vi "Select Active Channels.vi"(8 "error in (no error)":errorcluster, 10 "Active Channel(s)":T1[](array[typedef]), 11 "DPO4104 in":refnum<class "DPO4104.lvclass">) -> (0 "error out":errorcluster, 3 "DPO4104 out":refnum<class "DPO4104.lvclass">)   [LabVIEW 2018, in "DPO4104.lvlib" / "DPO4104.lvclass"]
doc: "This Override method is used to set active channels for the Oscope. Use the 'Active Channel(s)' control to select channel(s)."
uses:
  DPO4104.lvclass
  PPLs/Oscilloscope/Parent/Oscilloscope.lvlibp/Custom Controls/Analog Channels.ctl
  PPLs/Oscilloscope/Parent/Oscilloscope.lvlibp/Oscilloscope.lvclass
  C:/Projects/LabVIEW/PPLs/Oscilloscope/Parent/Oscilloscope.lvlibp/Oscilloscope.lvclass
  PPLs/Oscilloscope/Parent/Oscilloscope.lvlibp
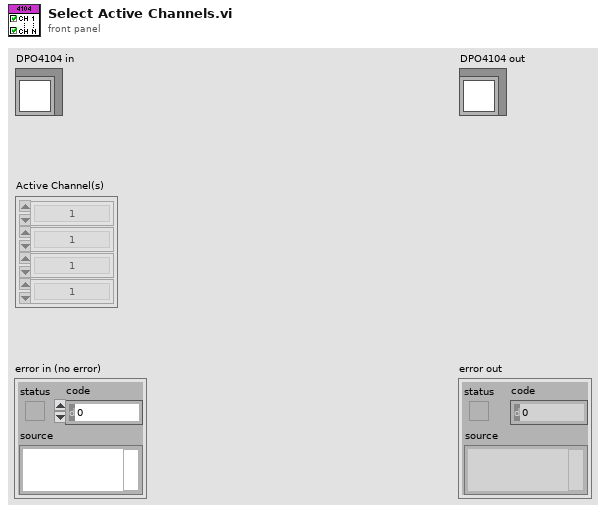
[diagram p1: front panel]
types:
  T1 = typedef "Oscilloscope.lvlibp/Analog Channels.ctl" = enum16{"1", "2", "3", "4", "5", "6", "7", "8", "9", "10", "11", "12", "13", "14", "15", "16"}
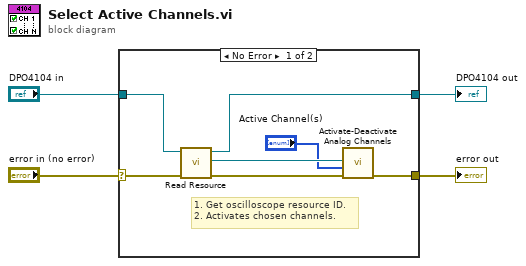
[diagram p0: block diagram]
diagram:
  n1 = case shown="No Error" "error in (no error)" {
    selector: "error in (no error)" -> [w10 w13]
    tunnel: [w6 w13] -> w3
    tunnel: "DPO4104 in" -> [w11 w12]
    tunnel: [w9 w12] -> w1
    frame No Error {
      # "1. Get oscilloscope resource ID.\n2. Activates chosen channels."
      n2 = call "Read Resource.vi"("error in (no error)"=w10, "Oscilloscope in"=w11) -> ("error out"=w7:errorcluster, "Resource"=w8:refnum<visa-resource-name>, "Oscilloscope out"=w9:refnum<class "DPO4104.lvclass">)  [unwired: 7 in]
      n3 = call "Activate-Deactivate Analog Channels.vi"("error in (no error)"=w7, "Active Channel(s)"="Active Channel(s)", "VISA resource name"=w8) -> ("error out"=w6:errorcluster)  [unwired: 7 in, 1 out]
    }
    frame Error {
    }
  }
  "error out" <- w3
  "DPO4104 out" <- w1
